vi "Conseguir_bits_digitales.vi"(11 "element":u32) -> (1 "Boolean 2":bool, 2 "Boolean 3":bool, 3 "Boolean 4":bool, 4 "Boolean":bool)   [LabVIEW 2024]
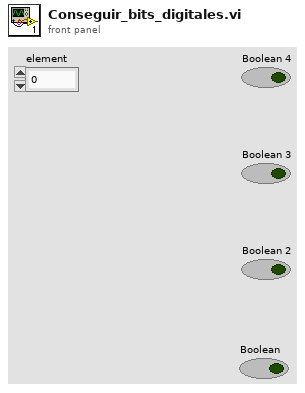
[diagram p1: front panel]
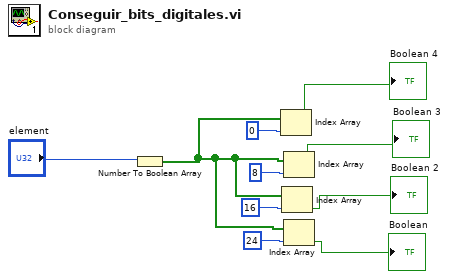
[diagram p0: block diagram]
diagram:
  n1 = Number To Boolean Array(number="element") -> (Boolean array=w7:bool[])
  n2 = Index Array(array=w7, index=0) -> (element=→"Boolean 4":bool)
  n3 = Index Array(array=w7, index=16) -> (element=→"Boolean 2":bool)
  n4 = Index Array(array=w7, index=8) -> (element=→"Boolean 3":bool)
  n5 = Index Array(array=w7, index=24) -> (element=→"Boolean":bool)
